vi "RFmxSpecAn Get Results Guts Deployed(Harms).vi"(0 "Refnum in":T1, 5 "Center Freq (Hz)":dbl, 11 "error in (no error)":errorcluster) -> (4 "Refnum out":T1, 6 "Peak Frequency (Hz)":dbl format="%.6p", 8 "Peak Amplitude":dbl format="%.2f", 15 "error out":errorcluster)   [LabVIEW 2018]
uses:
  <vilib>/RFmx/RFInstr/mx/Support/RFmxInstrSupport.llb/niRFmx Instrument Handle.ctl
  <vilib>/RFmx/SpecAn/mx/RFmxSpecAn.llb/RFmxSpecAn Spectrum Fetch Measurement.vi
  <resource>/objmgr/RFmxSpecAn.rc
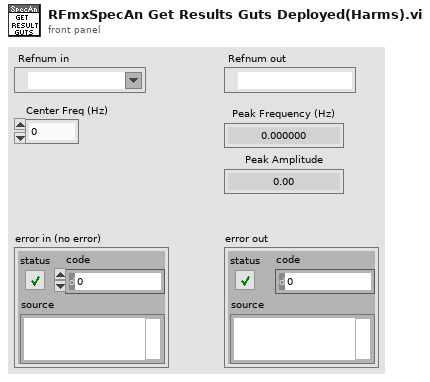
[diagram p1: front panel]
types:
  T1 = typedef "niRFmx Instrument Handle.ctl" = refnum<k21>
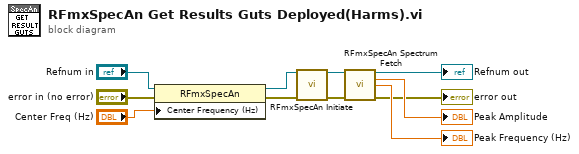
[diagram p0: block diagram]
diagram:
  n1 = property class="RFmxSpecAn"(reference="Refnum in", error in="error in (no error)", "Center Frequency (Hz)"="Center Freq (Hz)") -> (reference out=w6:T1, error out=w5:errorcluster)
  n2 = call <vilib>:"RFmxSpecAn Initiate.vi"("Instrument Handle In"=w6, "error in (no error)"=w5) -> ("Instrument Handle Out"=w3:refnum<k21>, "error out"=w4:errorcluster)  [unwired: 11 in, 1 out]
  n3 = call-poly <vilib>:"RFmxSpecAn Spectrum Fetch.vi"("Instrument Handle In"=w3, "error in (no error)"=w4) -> ("Instrument Handle Out"=→"Refnum out":refnum<k21>, "Peak Amplitude"=→"Peak Amplitude":dbl, "Peak Frequency (Hz)"=→"Peak Frequency (Hz)":dbl, "error out"=→"error out":errorcluster)  [unwired: 9 in, 1 out]
